vi "FillScanFuncTreeV2.vi"(6 "AddSymbol(True)":bool=TRUE, 7 "Multi ScanPar":bool[](array[boolean]), 8 "ErrorIn(No Error)":errorcluster caption="entrée d'erreur (pas d'erreur)", 9 "Active ScanPar":bool[](array[boolean]), 10 "ScanFunc":string[][](array[string]), 11 "ScanTreeRef":refnum<vi>) -> (0 "sortie d'erreur":errorcluster, 1 "Active ScanParOut":bool[](array[boolean]), 5 "Multi ScanParOut":bool[](array[boolean]))   [LabVIEW 2019]
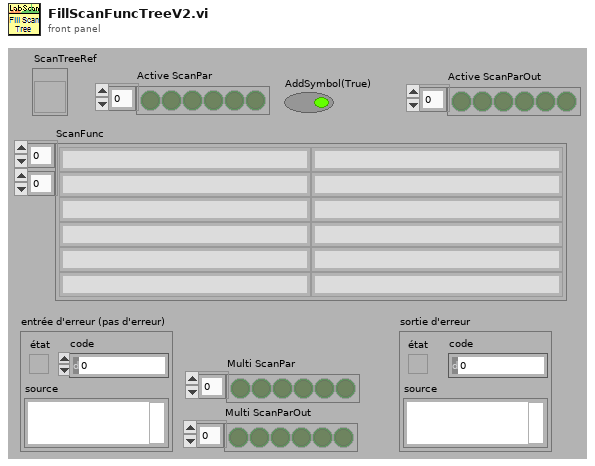
[diagram p1: front panel]
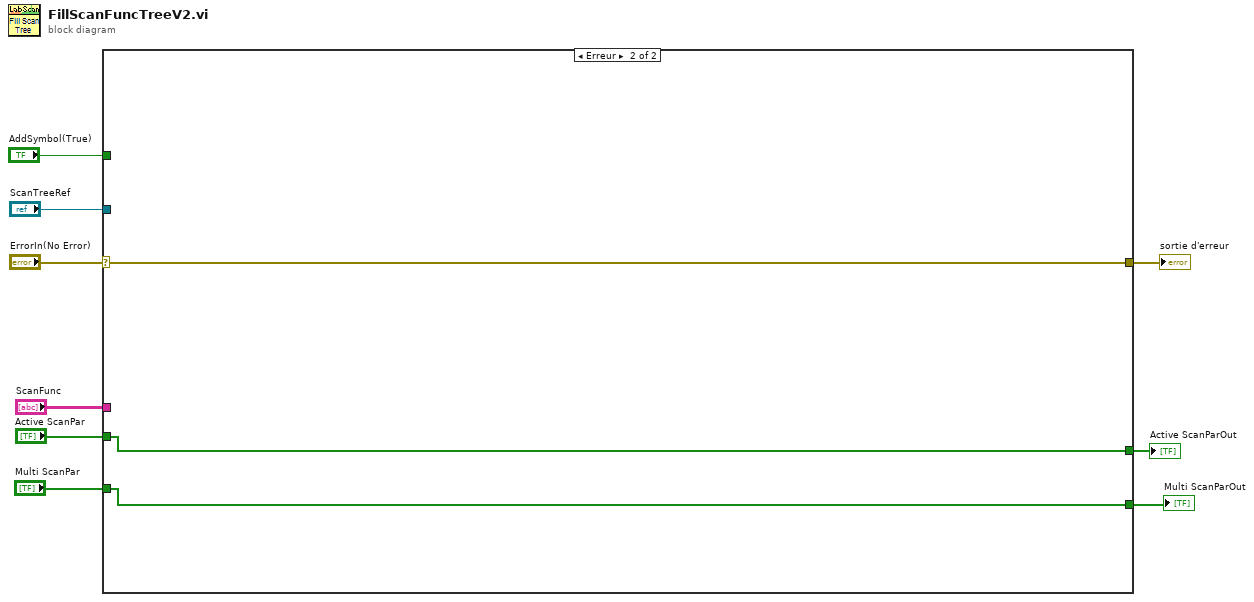
[diagram p0: block diagram]
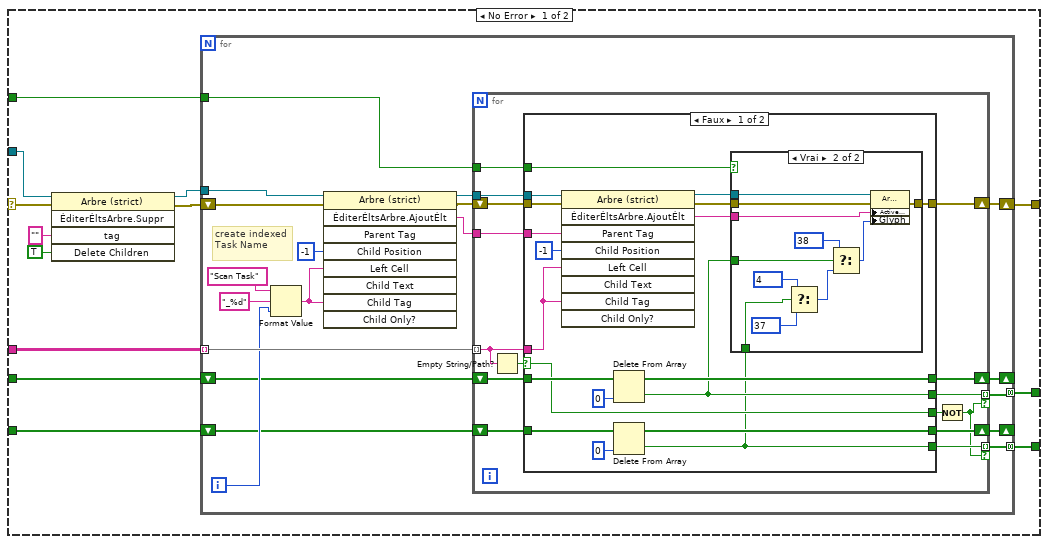
[diagram p2: hidden frame]
diagram:
  n1 = case shown="Erreur" "ErrorIn(No Error)" {
    selector: "ErrorIn(No Error)" -> [w20 w94]
    tunnel: [w21 w94] -> w8
    tunnel: "ScanFunc" -> [w22 _]
    tunnel: "ScanTreeRef" -> [w19 _]
    tunnel: "Active ScanPar" -> [w14 w93]
    tunnel: "AddSymbol(True)" -> [w13 _]
    tunnel: [w12 w93] -> w3
    tunnel: "Multi ScanPar" -> [w11 w92]
    tunnel: [w10 w92] -> w1
    frame No Error {
      n2 = invoke on="Nœud de méthode" class="Arbre (strict)" method="ÉditerÉltsArbre.Suppr"(reference=w19, error in=w20, "tag"="" ("Tag"), "Delete Children"=TRUE ("Supprimer les enfants ?")) -> (reference out=w18:refnum<vi>, error out=w17:errorcluster)  [unwired: 1 in, 3 out]
      n3 = for {
        tunnel: w22 -> [w41] mode=indexing
        tunnel: w18 -> [w30]
        shift-right: [w32] -> w21
        shift-left: w17 -> [w37]
        shift-right: [w28] -> _
        shift-left: w14 -> [w29]
        tunnel: w13 -> [w27]
        tunnel: [w26] -> w12 mode=concatenating
        shift-right: [w24] -> _
        shift-left: w11 -> [w25]
        tunnel: [w23] -> w10 mode=concatenating
        i -> [w38]
        # "create indexed Task Name"
        n4 = Format Value(string ("")="Scan Task" ("ClassName"), format string="_%d" ("chaîne de format"), value (0)=w38) -> (output string=w36:string)
        n5 = invoke on="Nœud de méthode" class="Arbre (strict)" method="ÉditerÉltsArbre.AjoutÉlt"(reference=w30, error in=w37, "Child Position"=-1 ("Position de l'enfant"), "Left Cell"=w36, "Child Tag"=w36) -> (reference out=w35:refnum<vi>, error out=w34:errorcluster, "Edit Tree Items:Add Item"=w33:string)  [unwired: 4 in, 6 out]
        n6 = for {
          tunnel: w41 -> [w51] mode=indexing
          tunnel: w35 -> [w56]
          tunnel: w33 -> [w54]
          shift-right: [w53] -> w32
          shift-left: w34 -> [w55]
          shift-right: [w49] -> w28
          shift-left: w29 -> [w50]
          tunnel: w27 -> [w48]
          tunnel: [w47] -> w26 mode=indexing if=w42
          shift-right: [w44] -> w24
          shift-left: w25 -> [w45]
          tunnel: [w43] -> w23 mode=indexing if=w42
          n7 = Empty String/Path?(string/path=w51) -> (empty?=w52:bool)
          n8 = case shown="Faux" w52 {
            selector: w52 -> [w61 w89]
            tunnel: w51 -> [w71 _]
            tunnel: w56 -> [w75 _]
            tunnel: w55 -> [w74 w91]
            tunnel: w54 -> [w73 _]
            tunnel: [w68 w91] -> w53
            tunnel: w50 -> [w66 w90]
            tunnel: [w64 w90] -> w49
            tunnel: w48 -> [w63 _]
            tunnel: [w62 _] -> w47
            tunnel: [w61 w89] -> w46
            tunnel: w45 -> [w59 w88]
            tunnel: [w58 w88] -> w44
            tunnel: [w57 _] -> w43
            frame False {
              n9 = invoke on="Nœud de méthode" class="Arbre (strict)" method="ÉditerÉltsArbre.AjoutÉlt"(reference=w75, error in=w74, "Parent Tag"=w73, "Child Position"=-1 ("Position de l'enfant"), "Left Cell"=w71, "Child Tag"=w71) -> (reference out=w70:refnum<vi>, error out=w69:errorcluster, "Edit Tree Items:Add Item"=w67:string)  [unwired: 3 in, 6 out]
              n10 = Delete From Array(array=w66, index=0 ("indice")) -> (deleted portion=w62:bool, array with subset deleted=w64:bool[])  [unwired: 1 in]
              n11 = Delete From Array(array=w59, index=0 ("indice")) -> (deleted portion=w57:bool, array with subset deleted=w58:bool[])  [unwired: 1 in]
              n12 = case shown="Vrai" w63 {
                tunnel: w70 -> [_ w87]
                tunnel: w69 -> [w76 w86]
                tunnel: [w76 w85] -> w68
                tunnel: w67 -> [_ w84]
                tunnel: w62 -> [_ w82]
                tunnel: w57 -> [_ w80]
                frame False {
                }
                frame True {
                  n13 = Select(t=4 ("symboles"), s=w80, f=37 ("symboles")) -> (s? t:f=w77:i32)
                  n14 = Select(t=38 ("symboles"), s=w82, f=w77) -> (s? t:f=w81:i32)
                  n15 = property class="Arbre (strict)"(reference=w87, error in=w86, "Active Item Tag"=w84, "Glyph"=w81) -> (error out=w85:errorcluster)  [unwired: 1 out]
                }
              }
            }
            frame True {
              # "Chaine vide: ne pas ajouter"
            }
          }
          n16 = Not(x=w46) -> (.not. x?=w42:bool)
        }
      }
    }
    frame Error {
    }
  }
  "sortie d'erreur" <- w8
  "Active ScanParOut" <- w3
  "Multi ScanParOut" <- w1
